vi "Launch New Connection Handler.vi"(8 "error in (no error)":errorcluster, 10 "Connection":refnum<class "IConnection.lvclass">, 11 "Network Session Handler in":refnum<class "Network Session Handler.lvclass">) -> (0 "error out":errorcluster, 2 "Loop Timeout":i32, 3 "Network Session Handler out":refnum<class "Network Session Handler.lvclass">)   [LabVIEW 2019, in "Network Interface.lvlib" / "Network Session Handler.lvclass"]
uses:
  <vilib>/gpm_packages/@cs/Network-Sink/Source/Network Interface/Network Session Handler/Network Session Handler.lvclass
  <vilib>/gpm_packages/@cs/Network-Sink/Source/Network Interface/IConnection/IConnection.lvclass
  <vilib>/gpm_packages/@cs/Network-Sink/Source/Network Interface/Network Session Handler/Network Session Handler.lvclass/Network Session Handler.ctl
  <vilib>/gpm_packages/@cs/Network-Sink/Source/Network Interface/IConnection/IConnection.lvclass/IConnection.ctl
  <vilib>/gpm_packages/@cs/Network-Sink/Source/Network Interface/Network Session Handler/Connection Handler.ctl
  <vilib>/gpm_packages/@cs/Network-Sink/Source/Network Interface/Message Queue/Message Queue.lvclass
  <vilib>/gpm_packages/@cs/event-logger/Source/Composed Log/Types/Log Level.ctl
  <vilib>/gpm_packages/@cs/event-logger/Source/Composed Log/LoggerReference/LoggerReference.lvclass/LoggerReference.ctl
  <vilib>/gpm_packages/@cs/event-logger/Source/Composed Log/LoggerReference/Log.vi
  <vilib>/gpm_packages/@cs/event-logger/Source/Composed Log/LoggerReference/Get Valid Event Time.vi
  <vilib>/gpm_packages/@cs/event-logger/Source/Composed Log/LoggerReference/Remove Stale Logs.vi
  <vilib>/gpm_packages/@cs/Network-Sink/Source/Network Interface/Connection Handler/Connection Handler.lvclass
  <vilib>/gpm_packages/@cs/event-logger/Source/Composed Log/Composed Log.lvlib
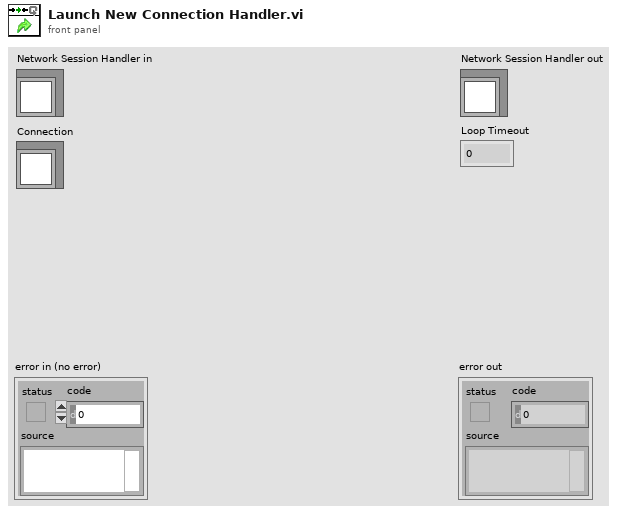
[diagram p1: front panel]
types:
  T1 = typedef "Network Interface.lvlib/Network Session Handler.lvclass/Connection Handler.ctl" = cluster{"ID":string, "Handler Queue":refnum<class "Message Queue.lvclass">}
  T2 = typedef "Composed Log.lvlib/Log Level.ctl" = enum16{"Debug", "Info", "Warning", "Error", "Critical"}
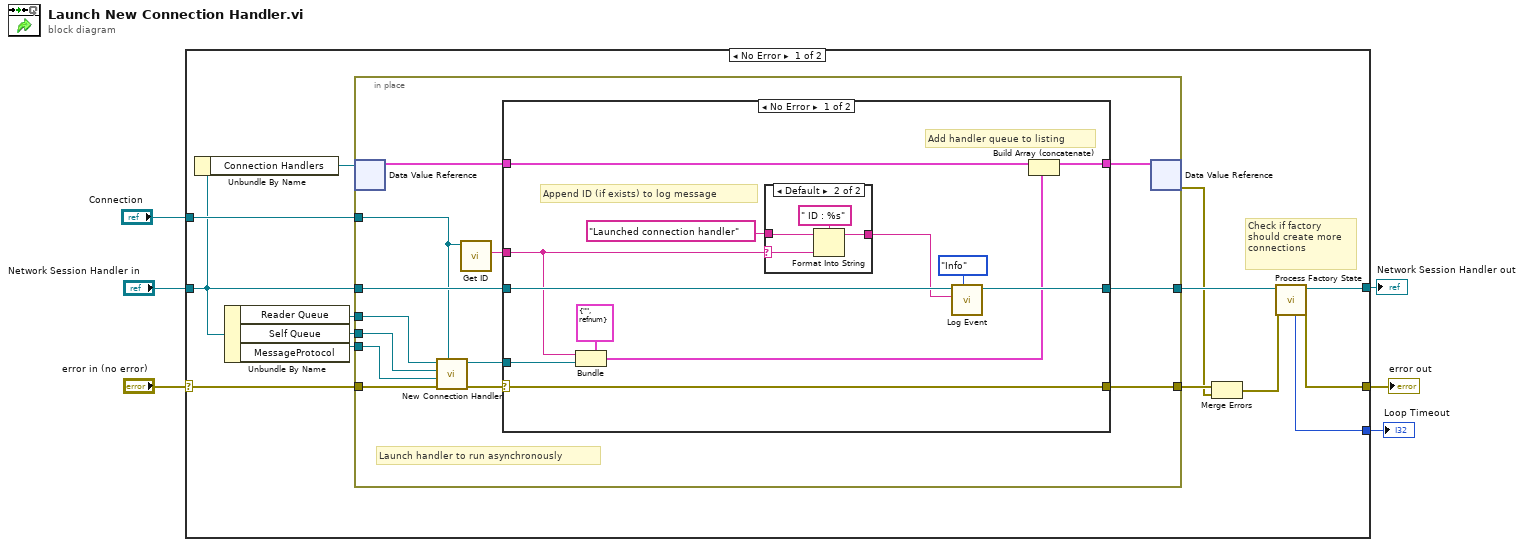
[diagram p0: block diagram]
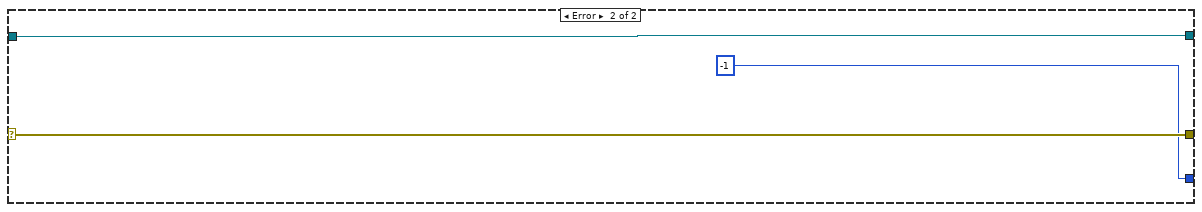
[diagram p4: hidden frame]
diagram:
  n1 = case shown="No Error" "error in (no error)" {
    selector: "error in (no error)" -> [w20 w55]
    tunnel: "Connection" -> [w14 _]
    tunnel: "Network Session Handler in" -> [w7 w56]
    tunnel: [w18 w56] -> w3
    tunnel: [w16 w55] -> w2
    tunnel: [w15 -1 ("Loop Timeout")] -> w1
    frame No Error {
      # "Check if factory should create more connections"
      n2 = Unbundle By Name(w7) -> ("Connection Handlers"=w13:refnum<data-value>)
      n3 = Unbundle By Name(w7) -> ("Reader Queue"=w10:refnum<queue>, "Self Queue"=w9:refnum<class "Message Queue.lvclass">, "MessageProtocol"=w8:refnum<class "IMessagingProtocol.lvclass">)
      n4 = in-place {
        in-place-border: w20 -> [w33]
        in-place-border: w7 -> [w32]
        in-place-border: [w29] -> w19
        in-place-border: [w28] -> w17
        in-place-border: w14 -> [w26]
        in-place-border: w10 -> [w23]
        in-place-border: w9 -> [w22]
        in-place-border: w8 -> [w21]
        # "Launch handler to run asynchronously"
        n5 = in-place-dvr #1(w13) -> (w25:T1[])  [unwired: 1 out]
        n6 = call <vilib>:"New Connection Handler.vi"("Connection"=w26, "error in"=w33, "Message Protocol"=w21, "Controller Queue"=w22, "Read Queue"=w23) -> ("error out"=w31:errorcluster, "Handler Queue"=w30:refnum<class "Message Queue.lvclass">)  [unwired: 5 in]
        n7 = call <vilib>:"Get ID.vi"("IConnection in"=w26) -> ("ID"=w27:string)  [unwired: 10 in]
        n8 = case shown="No Error" w31 {
          selector: w31 -> [w45 w52]
          tunnel: w32 -> [w44 w53]
          tunnel: [w37 w53] -> w29
          tunnel: w30 -> [w40 _]
          tunnel: [w45 w52] -> w28
          tunnel: w27 -> [w39 _]
          tunnel: w25 -> [w36 w51]
          tunnel: [w35 w51] -> w24
          frame No Error {
            # "Append ID (if exists) to log message"
            # "Add handler queue to listing"
            n9 = Bundle(cluster=T1 {"ID"="", "Handler Queue"=refnum}, "ID"=w39, "Handler Queue"=w40) -> (w34:T1)
            n10 = case shown="Default" w39 {
              selector: w39 -> [_ w49]
              tunnel: "Launched connection handler" ("Event") -> [w46 w48]
              tunnel: [w46 w50] -> w41
              frame "" {
              }
              frame Default {
                n11 = Format Into String(format string=" ID : %s", initial string=w48, w49) -> (resulting string=w50:string)  [unwired: 1 in, 1 out]
              }
            }
            n12 = call <vilib>:"Log Event.vi"("Event Level"=Log_Level."Info", "Event"=w41, "Network Session Handler in"=w44) -> ("Network Session Handler out"=w37:refnum<class "Network Session Handler.lvclass">)  [unwired: 7 in, 1 out]
            n13 = Build Array (concatenate)(w36, w34) -> (w35:T1[])
          }
          frame Error {
          }
        }
        n14 = in-place-dvr #1(w24) -> (w11:errorcluster)  [unwired: 1 out]
      }
      n15 = Merge Errors(w17, w11) -> (w12:errorcluster)
      n16 = call <vilib>:"Process Factory State.vi"("error in (no error)"=w12, "Network Session Handler in"=w19) -> ("error out"=w16:errorcluster, "Network Session Handler out"=w18:refnum<class "Network Session Handler.lvclass">, "Loop Timeout"=w15:i32)  [unwired: 7 in]
    }
    frame Error {
    }
  }
  "error out" <- w2
  "Network Session Handler out" <- w3
  "Loop Timeout" <- w1
